vi "PPMS.getAll.vi"(8 "error in (no error)":errorcluster, 11 "instrument.PPMS2 in":refnum<class "instrument.PPMS2.lvclass">) -> (0 "error out":errorcluster, 2 "getAll":T1, 3 "instrument.PPMS2 out":refnum<class "instrument.PPMS2.lvclass">)   [LabVIEW 2019, in "instrument.PPMS2.lvclass"]
uses:
  instrument.PPMS2.lvclass
  C:/Users/patrick/Documents/GitHub/PPMS-Monitor-and-Control/lvsrc/instrument.PPMS/instrument.PPMS.lvclass
  instrument.PPMS/Typedefs/PPMS.getAll--cluster.ctl
  instrument.PPMS/instrument.PPMS.lvclass/instrument.PPMS.ctl
  instrument.PPMS/instrument.PPMS.lvclass
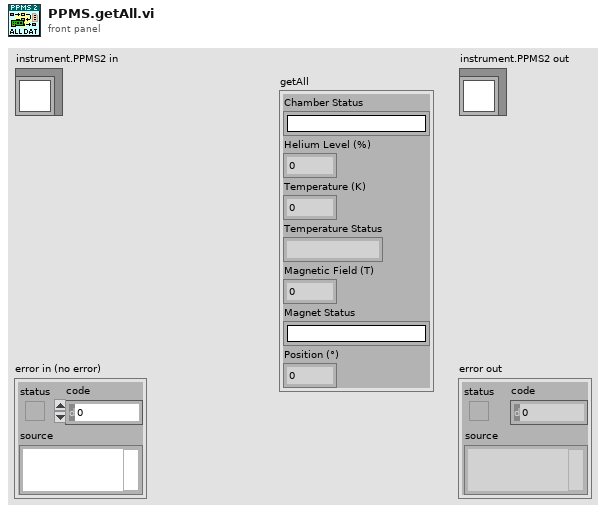
[diagram p1: front panel]
types:
  T1 = typedef "instrument.PPMS.lvclass/PPMS.getAll--cluster.ctl" = cluster{"Chamber Status":string, "Helium Level (%)":dbl, "Temperature (K)":dbl, "Temperature Status":string, "Magnetic Field (T)":dbl, "Magnet Status":string, "Position (°)":dbl}
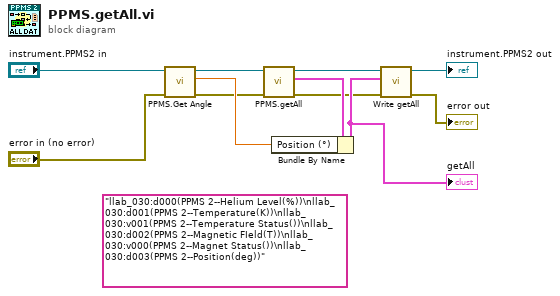
[diagram p0: block diagram]
diagram:
  (unwired) "llab_030:d000(PPMS 2--Helium Level(%))\nllab_030:d001(PPMS 2--Temperature(K))\nllab_030:v001(PPMS 2--Temperature Status())\nllab_030:d002(PPMS 2--Magnetic FIeld(T))\nllab_030:v000(PPMS 2--Magnet Status())\nllab_030:d003(PPMS 2--Position(deg))" ("Paths")
  n1 = call "PPMS.Get Angle.vi"("error in (no error)"="error in (no error)", "instrument.PPMS"="instrument.PPMS2 in") -> ("error out"=w4:errorcluster, "Angle (°)"=w11:dbl, "instrument.PPMS out"=w3:refnum<class "instrument.PPMS2.lvclass">)  [unwired: 7 in]
  n2 = call-parent "PPMS.getAll.vi"("error in (no error)"=w4, "instrument.PPMS in"=w3) -> ("error out"=w5:errorcluster, "getAll"=w8:T1, "instrument.PPMS out"=w6:refnum<class "instrument.PPMS2.lvclass">)  [unwired: 7 in]
  n3 = Bundle By Name(cluster=w8, "Position (°)"=w11) -> (w7:T1)
  "getAll" <- w7
  n4 = call "Write getAll.vi"("error in (no error)"=w5, "getAll"=w7, "instrument.PPMS in"=w6) -> ("error out"=→"error out":errorcluster, "instrument.PPMS out"=→"instrument.PPMS2 out":refnum<class "instrument.PPMS2.lvclass">)  [unwired: 7 in]
